vi "programa 3 pulsador.vi"() -> ()   [LabVIEW 2011]
panel:
  out "Boolean":bool
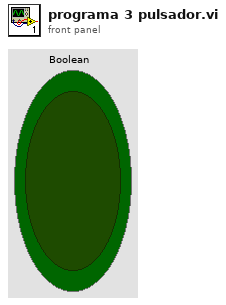
[diagram p1: front panel]
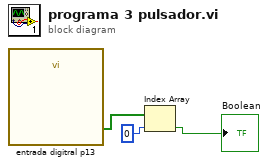
[diagram p0: block diagram]
diagram:
  n1 = call "entrada digitral p13"() -> ("data"=w2:bool[])  [unwired: 17 in, 2 out]
  n2 = Index Array(array=w2, index=0) -> (element=→"Boolean":bool)
